vi "Read U16.vi"(0 "I2C In":refnum<class "I2C.lvclass">, 1 "Slave Address":u8, 5 "Register":u32, 11 "Error In":errorcluster, 12 "Register Size":T2, 13 "Byte Order":T1) -> (4 "I2C Out":refnum<class "I2C.lvclass">, 6 "Value":u16, 15 "Error Out":errorcluster)   [LabVIEW 2020, in "lv_i2c_hal.lvlib" / "I2C.lvclass"]
uses:
  I2C.lvclass
  Register Address Size.ctl
  Byte Order.ctl
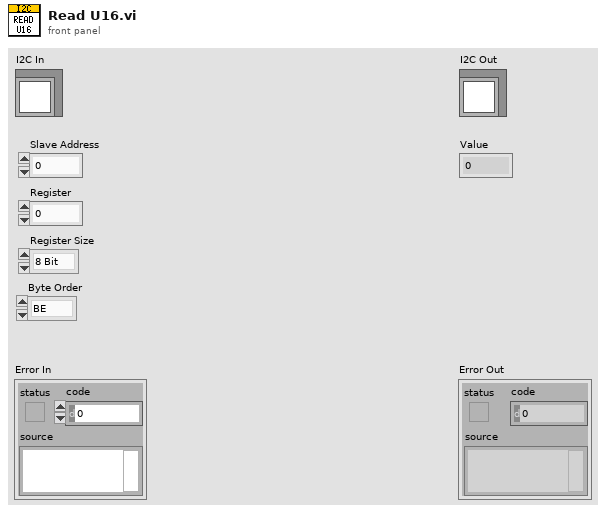
[diagram p1: front panel]
types:
  T1 = typedef "lv_i2c_hal.lvlib/I2C.lvclass/Byte Order.ctl" = enum16{"BE", "LE"}
  T2 = typedef "lv_i2c_hal.lvlib/I2C.lvclass/Register Address Size.ctl" = enum16{"8 Bit", "16 Bit", "24 Bit", "32 Bit"}
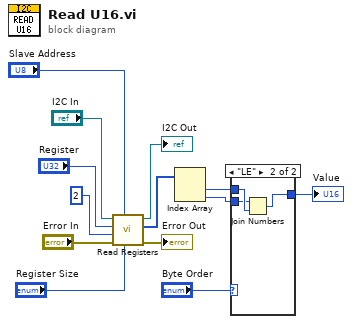
[diagram p0: block diagram]
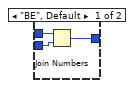
[diagram p2: hidden frame]
diagram:
  n1 = call "Read Registers.vi"("Register Size"="Register Size", "Slave Address"="Slave Address", "Error In"="Error In", "Count"=2, "Register"="Register", "I2C In"="I2C In") -> ("Error Out"=→"Error Out":errorcluster, "Values"=w10:u8[], "I2C Out"=→"I2C Out":refnum<class "I2C.lvclass">)  [unwired: 3 in]
  n2 = Index Array(array=w10) -> (element #1=w3:u8, element #2=w2:u8)  [unwired: 2 in]
  n3 = case shown="\"LE\"" "Byte Order" {
    tunnel: w3 -> [w16 w19]
    tunnel: w2 -> [w15 w18]
    tunnel: [w14 w17] -> w1
    frame "BE", Default {
      n4 = Join Numbers(hi=w16, lo=w15) -> ((hi.lo)=w14:u16)
    }
    frame "LE" {
      n5 = Join Numbers(hi=w18, lo=w19) -> ((hi.lo)=w17:u16)
    }
  }
  "Value" <- w1
